vi "pid-auto-tune.vi"() -> ()   [LabVIEW 2019]
uses:
  <vilib>/Rock Robotics/WPI/ThirdParty/JAS_Junk/TrajLib/TypeDef/PID_CONTROLLER.ctl
  <vilib>/Rock Robotics/WPI/ThirdParty/JAS_Junk/TrajLib/LinearFilter_ResetToValue.vi
  <vilib>/Rock Robotics/WPI/ThirdParty/JAS_Junk/TrajLib/LinearFilter_Calculate.vi
  <vilib>/Rock Robotics/WPI/ThirdParty/JAS_Junk/TrajLib/MathUtil_Clamp.vi
  <vilib>/Rock Robotics/WPI/ThirdParty/JAS_Junk/TrajLib/SlewRateLimiter_New.vi
  <vilib>/Rock Robotics/WPI/ThirdParty/JAS_Junk/TrajLib/SlewRateLimiter_Reset.vi
  <vilib>/Rock Robotics/WPI/ThirdParty/JAS_Junk/TrajLib/SlewRateLimiter_Calculate.vi
  <vilib>/Rock Robotics/WPI/ThirdParty/JAS_Junk/TrajLib/SlewRateLimiter_SetRate.vi
  <vilib>/Rock Robotics/WPI/ThirdParty/JAS_Junk/TrajLib/PIDController_AtSetpoint.vi
  <vilib>/Rock Robotics/WPI/ThirdParty/JAS_Junk/TrajLib/PIDController_SetPIDF.vi
  <vilib>/Rock Robotics/WPI/ThirdParty/JAS_Junk/TrajLib/PIDController_SetDerivativeFilter.vi
  <vilib>/Rock Robotics/WPI/ThirdParty/JAS_Junk/TrajLib/PIDController_SetIntegratorRange.vi
  <vilib>/Rock Robotics/WPI/ThirdParty/JAS_Junk/TrajLib/PIDController_SetTolerancePandV.vi
  <vilib>/Rock Robotics/WPI/ThirdParty/JAS_Junk/TrajLib/PIDController_DisableContinousInput.vi
  <vilib>/Rock Robotics/WPI/ThirdParty/JAS_Junk/TrajLib/PIDController_EnableContinousInput.vi
  <vilib>/Rock Robotics/WPI/ThirdParty/JAS_Junk/TrajLib/PIDController_Reset.vi
  <vilib>/Rock Robotics/WPI/ThirdParty/JAS_Junk/TrajLib/PIDController_New.vi
  <vilib>/Rock Robotics/WPI/ThirdParty/JAS_Junk/TrajLib/PIDController_SetOutputLimits.vi
  <vilib>/Rock Robotics/WPI/ThirdParty/JAS_Junk/TrajLib/PIDController_NewPeriod.vi
  <vilib>/Rock Robotics/SystemInterfaces/NetworkCommunication/NetComm_UsageReport_report.vi
  <vilib>/Rock Robotics/WPI/ThirdParty/JAS_Junk/TrajLib/Util_LibraryGlobals.vi
  <vilib>/Rock Robotics/WPI/ThirdParty/JAS_Junk/TrajLib/PIDController_AdvCalculate_FF_Sp_Pv.vi
  <vilib>/addons/control/pid/pid.llb/PID Lead-Lag (DBL).vi
  <vilib>/Rock Robotics/WPI/ThirdParty/JAS_Junk/TrajLib/LinearFilter_MovingAverage.vi
  <vilib>/Rock Robotics/WPI/ThirdParty/JAS_Junk/TrajLib/LinearFilter_LowPassBW1.vi
  <vilib>/Rock Robotics/WPI/ThirdParty/JAS_Junk/TrajLib/LinearFilter_LowPassBW2.vi
  <vilib>/Rock Robotics/WPI/ThirdParty/JAS_Junk/TrajLib/LinearFilter_HighPassBW1.vi
  <vilib>/Rock Robotics/WPI/ThirdParty/JAS_Junk/TrajLib/LinearFilter_HighPassBW2.vi
  <vilib>/addons/control/pid/NI_PID_pid.lvlib
  <vilib>/Rock Robotics/WPI/ThirdParty/JAS_Junk/TrajLib/Trajectory_Library.lvlib
panel:
  out "Plant and Test Data":T1
  out "Tuning Done":bool
  in  "Type of Controller":enum16{"P", "PI", "PID"}(ring)=enum."PI"
  in  "Controller Constant Type":T2(ring)=enum."Ziegler Nicols - Slow"
  in  "Procedure Type":enum16{"Open Loop Step", "Closed Loop Step"}(ring)
  out "New Tuning Parameters":T3
  out "Error Occured":bool
  in  "Tune":bool
  in  "CO Offset":dbl=0.25 format="%#_13g"
  out "Diagnostic Info":T4
  in  "Desired Speed":dbl(slide)=-0.22222222222222499 scale=-10.0..10.0 scale format="%#.1f"
  in  "Tab Control":T5(tab)
  in  "Enable Noise":bool=TRUE
  in  "Auto / Manual":bool=TRUE
  out "Dash Speed Demand":dbl format="%10.2f"
  out "Dash Speed Target":dbl format="%10.2f"
  out "DashLeft Wheel Speed":dbl(knob)=-2.895988890827539e-05 scale=-60.0..60.0
  out "Left Wheel ErrorFilt":dbl format="%11.3f"
  out "DashLeftMotorOutput":dbl format="%11.3f"
  out "Left Wheel Speed Filt":dbl format="%10.2f"
  out "Duration":dbl format="%11.3f"
  out "Late":dbl format="%11.3f"
  out "SP, PV, CO Left":T6(graph)
  in  "SetPoint Change Rate":dbl=80.0 min=1.0 max=9000.0 format="%14.4f"
  in  "Left Adv PID Limits":T7={"MaxInput"=50.0, "MinInput"=-50.0, "Continuous"=FALSE, "MaxOutput"=1.0, "MinOutput"=-1.0}
  in  "Left PID Error Tolerance":T8={"PositionTolerance"=0.001, "VelocityTolerance"=9.9e+30}
  in  "Left Adv PID Tuning":T9={"Kf"=0.02, "Kp"=0.06, "Ki"=0.1, "Kd"=0.004, "MaximumIntegral"=9.9e+30, "MinimumIntegral"=-9.9e+30, "Filter Derivative"=TRUE}
  out "Left PID Data":T10={"Kp"=0.0, "Ki"=0.0, "Kd"=0.0, "Period"=0.0, "Max_Integral"=0.0, "Min_Integral"=0.0, "Max_Input"=0.0, "Min_Input"=0.0, "Continuous"=FALSE, "PositionError"=0.0, "VelocityError"=0.0, "PrevError"=0.0, "TotalError"=0.0, "PositionTolerance"=0.0, "VelocityTolerance"=0.0, "SetPoint"=0.0, "Kf"=0.0, "Prev_Deriv"=0.0, "Prev_Deriv 2"=0.0, "DerivativeFilter"=FALSE, "Min_Output"=-9.99e+35, "Max_Output"=9.9e+35, "Prev_F_P"=0.0, "Prev_F_P_2"=0.0, "AntiWindupActive"=FALSE, "Measurement"=0.0} {"Measurement" format="%16_6e"; "Prev_F_P_2" format="%16_6e"; "Prev_F_P" format="%16_6e"; "Max_Output" format="%16_6e"; "Min_Output" format="%16_6e"; "Prev_Deriv 2" format="%16_6e"; "Prev_Deriv" format="%16_6e"; "Kf" format="%16_6e"; "SetPoint" format="%16_6e"; "VelocityTolerance" format="%16_6e"; "PositionTolerance" format="%16_6e"; "TotalError" format="%16_6e"; "PrevError" format="%16_6e"; "VelocityError" format="%16_6e"; "PositionError" format="%16_6e"; "Min_Input" format="%16_6e"; "Max_Input" format="%16_6e"; "Min_Integral" format="%16_6e"; "Max_Integral" format="%16_6e"; "Period" format="%16_6e"; "Kd" format="%16_6e"; "Ki" format="%16_6e"; "Kp" format="%16_6e"}
  in  "LeftWheelNoise":dbl
  out "LeftWheelSpeed":dbl
  out "LeftMotorOutput":dbl
  out "SpeedSetpoint":dbl
  in  "SpeedTarget":dbl
  in  "SpeedControlEnabled":bool
  out "LibUsage_Kinematics":i32 format="%20.0f"
  out "LibUsage_TrapezoidProfile":i32 format="%20.0f"
  out "LibUsage_LinearFIlter":i32 format="%20.0f"
  out "LibUsage_Odometry":i32 format="%20.0f"
  out "LibUsage_PIDController":i32 format="%20.0f"
  out "LibUsage_ProfiledPID":i32 format="%20.0f"
  # "Enter a desired speed and then press the Set Speed Target \nbutton.  This simulates the joystick input."
  # "FT/SEC"
  # "Example of Closed Loop Motor Speed Control\nUses Advanced PID"
  # "This value shows the current speed of each wheel.  This is measured by an encoder.  The encoder measures\n speed by counting pulses of the wheel turning and dividing by the time interval.  Total distance change\nis also a result.  This value is called the \"Process Variable\"."
  # "FT/SEC"
  # "FT/SEC"
  # "The Speed Target is rate limited so not to make\nto drastic a change in the desired speed.  (This is\nwhat happens mechanically when pushing the gas\npedal of a real car.)"
  # "This error value shows the error between the current speed\nand the speed demand."
  # "FT/SEC"
  # "This example adds a \"Manual\" mode so that the still operates\nif the encoder fails."
  # "FT/SEC"
  # "This value shows the current motor output demand.  This could also be a motor speed demand and \nanother closed loop controller would control the motor speed.  In this simple example this value is \nused to drive the simulated motor directly.  This motor demand is called the \"Control Output\"."
  # "Enables some simulated process noise"
  # "FT/SEC/SEC"
  # "These are the tuning parameters for the PID VI"
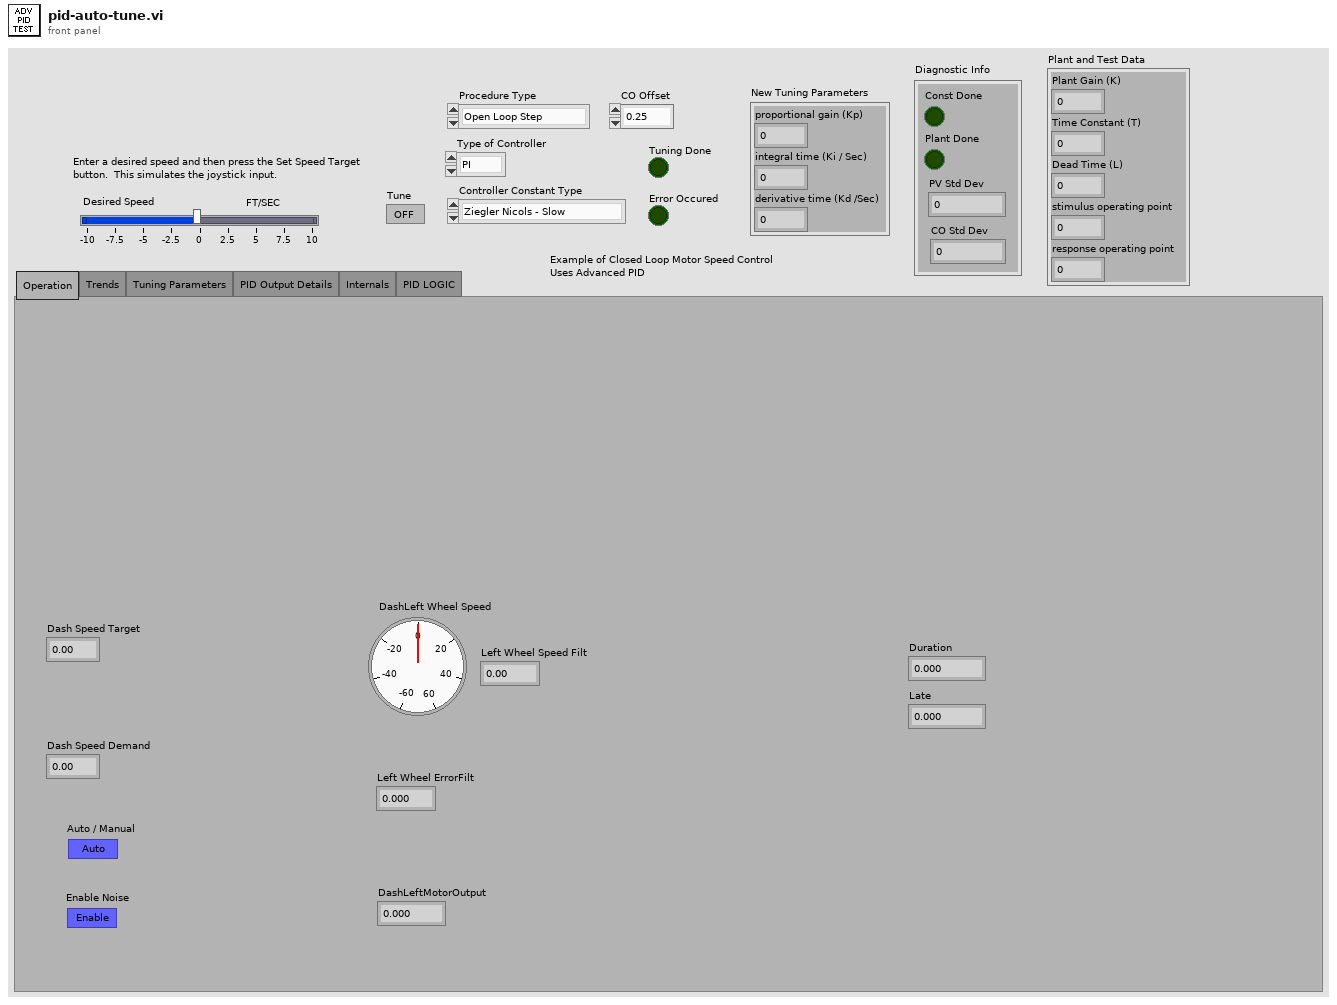
[diagram p1: front panel]
types:
  T1 = cluster{"Plant Gain (K)":dbl, "Time Constant (T)":dbl, "Dead Time (L)":dbl, "stimulus operating point":dbl, "response operating point":dbl}
  T2 = enum16{"Ziegler Nicols - Fast", "Ziegler Nicols - Normal", "Ziegler Nicols - Slow", "CHR regulator - 0% overshoot", "CHR regulator - 20% overshoot", "CHR servo - 0 % overshoot", "CHR servo - 20% overshoot"}
  T3 = cluster{"proportional gain (Kp)":dbl, "integral time (Ki / Sec)":dbl, "derivative time (Kd /Sec)":dbl}
  T4 = cluster{"Const Done":bool, "Plant Done":bool, "PV Std Dev":dbl, "CO Std Dev":dbl}
  T5 = enum32{"Operation", "Trends", "Tuning Parameters", "PID Output Details", "Internals", "PID LOGIC"}
  T6 = cluster{"MotorDemand":dbl, "CurrentSetpoint":dbl, "CurrentPosition":dbl}
  T7 = cluster{"MaxInput":dbl, "MinInput":dbl, "Continuous":bool, "MaxOutput":dbl, "MinOutput":dbl}
  T8 = cluster{"PositionTolerance":dbl, "VelocityTolerance":dbl}
  T9 = cluster{"Kf":dbl, "Kp":dbl, "Ki":dbl, "Kd":dbl, "MaximumIntegral":dbl, "MinimumIntegral":dbl, "Filter Derivative":bool}
  T10 = typedef "Trajectory_Library.lvlib/PID_CONTROLLER.ctl" = cluster{"Kp":dbl, "Ki":dbl, "Kd":dbl, "Period":dbl, "Max_Integral":dbl, "Min_Integral":dbl, "Max_Input":dbl, "Min_Input":dbl, "Continuous":bool, "PositionError":dbl, "VelocityError":dbl, "PrevError":dbl, "TotalError":dbl, "PositionTolerance":dbl, "VelocityTolerance":dbl, "SetPoint":dbl, "Kf":dbl, "Prev_Deriv":dbl, "Prev_Deriv 2":dbl, "DerivativeFilter":bool, "Min_Output":dbl, "Max_Output":dbl, "Prev_F_P":dbl, "Prev_F_P_2":dbl, "AntiWindupActive":bool, "Measurement":dbl}
  T11 = cluster{"gain":dbl, "lag time":dbl, "lead time":dbl}
  T12 = enum16{"Moving Average", "Low Pass 1st Order Butterworth", "Low Pass 2nd Order Butterworth", "High Pass 1st Order Butterworth", "High Pass 2nd Order Butterworth"}
  T13 = cluster{"LeftMotorOutput":dbl, "SpeedSetpoint":dbl, "LeftWheelSpeed":dbl}
  T14 = cluster{"Controller Constant Type":enum16{"Ziegler Nicols - Fast", "Ziegler Nicols - Normal", "Ziegler Nicols - Slow", "CHR regulator - 0% overshoot", "CHR regulator - 20% overshoot", "CHR servo - 0 % overshoot", "CHR servo - 20% overshoot"}, "Type of Controller":enum16{"P", "PI", "PID"}, "CO Offset":dbl, "Kn":dbl, "Tuning Tolerance":dbl, "Plant Tolerance":dbl, "Newest Avg Time ":i32, "Long Ave Time":i32}
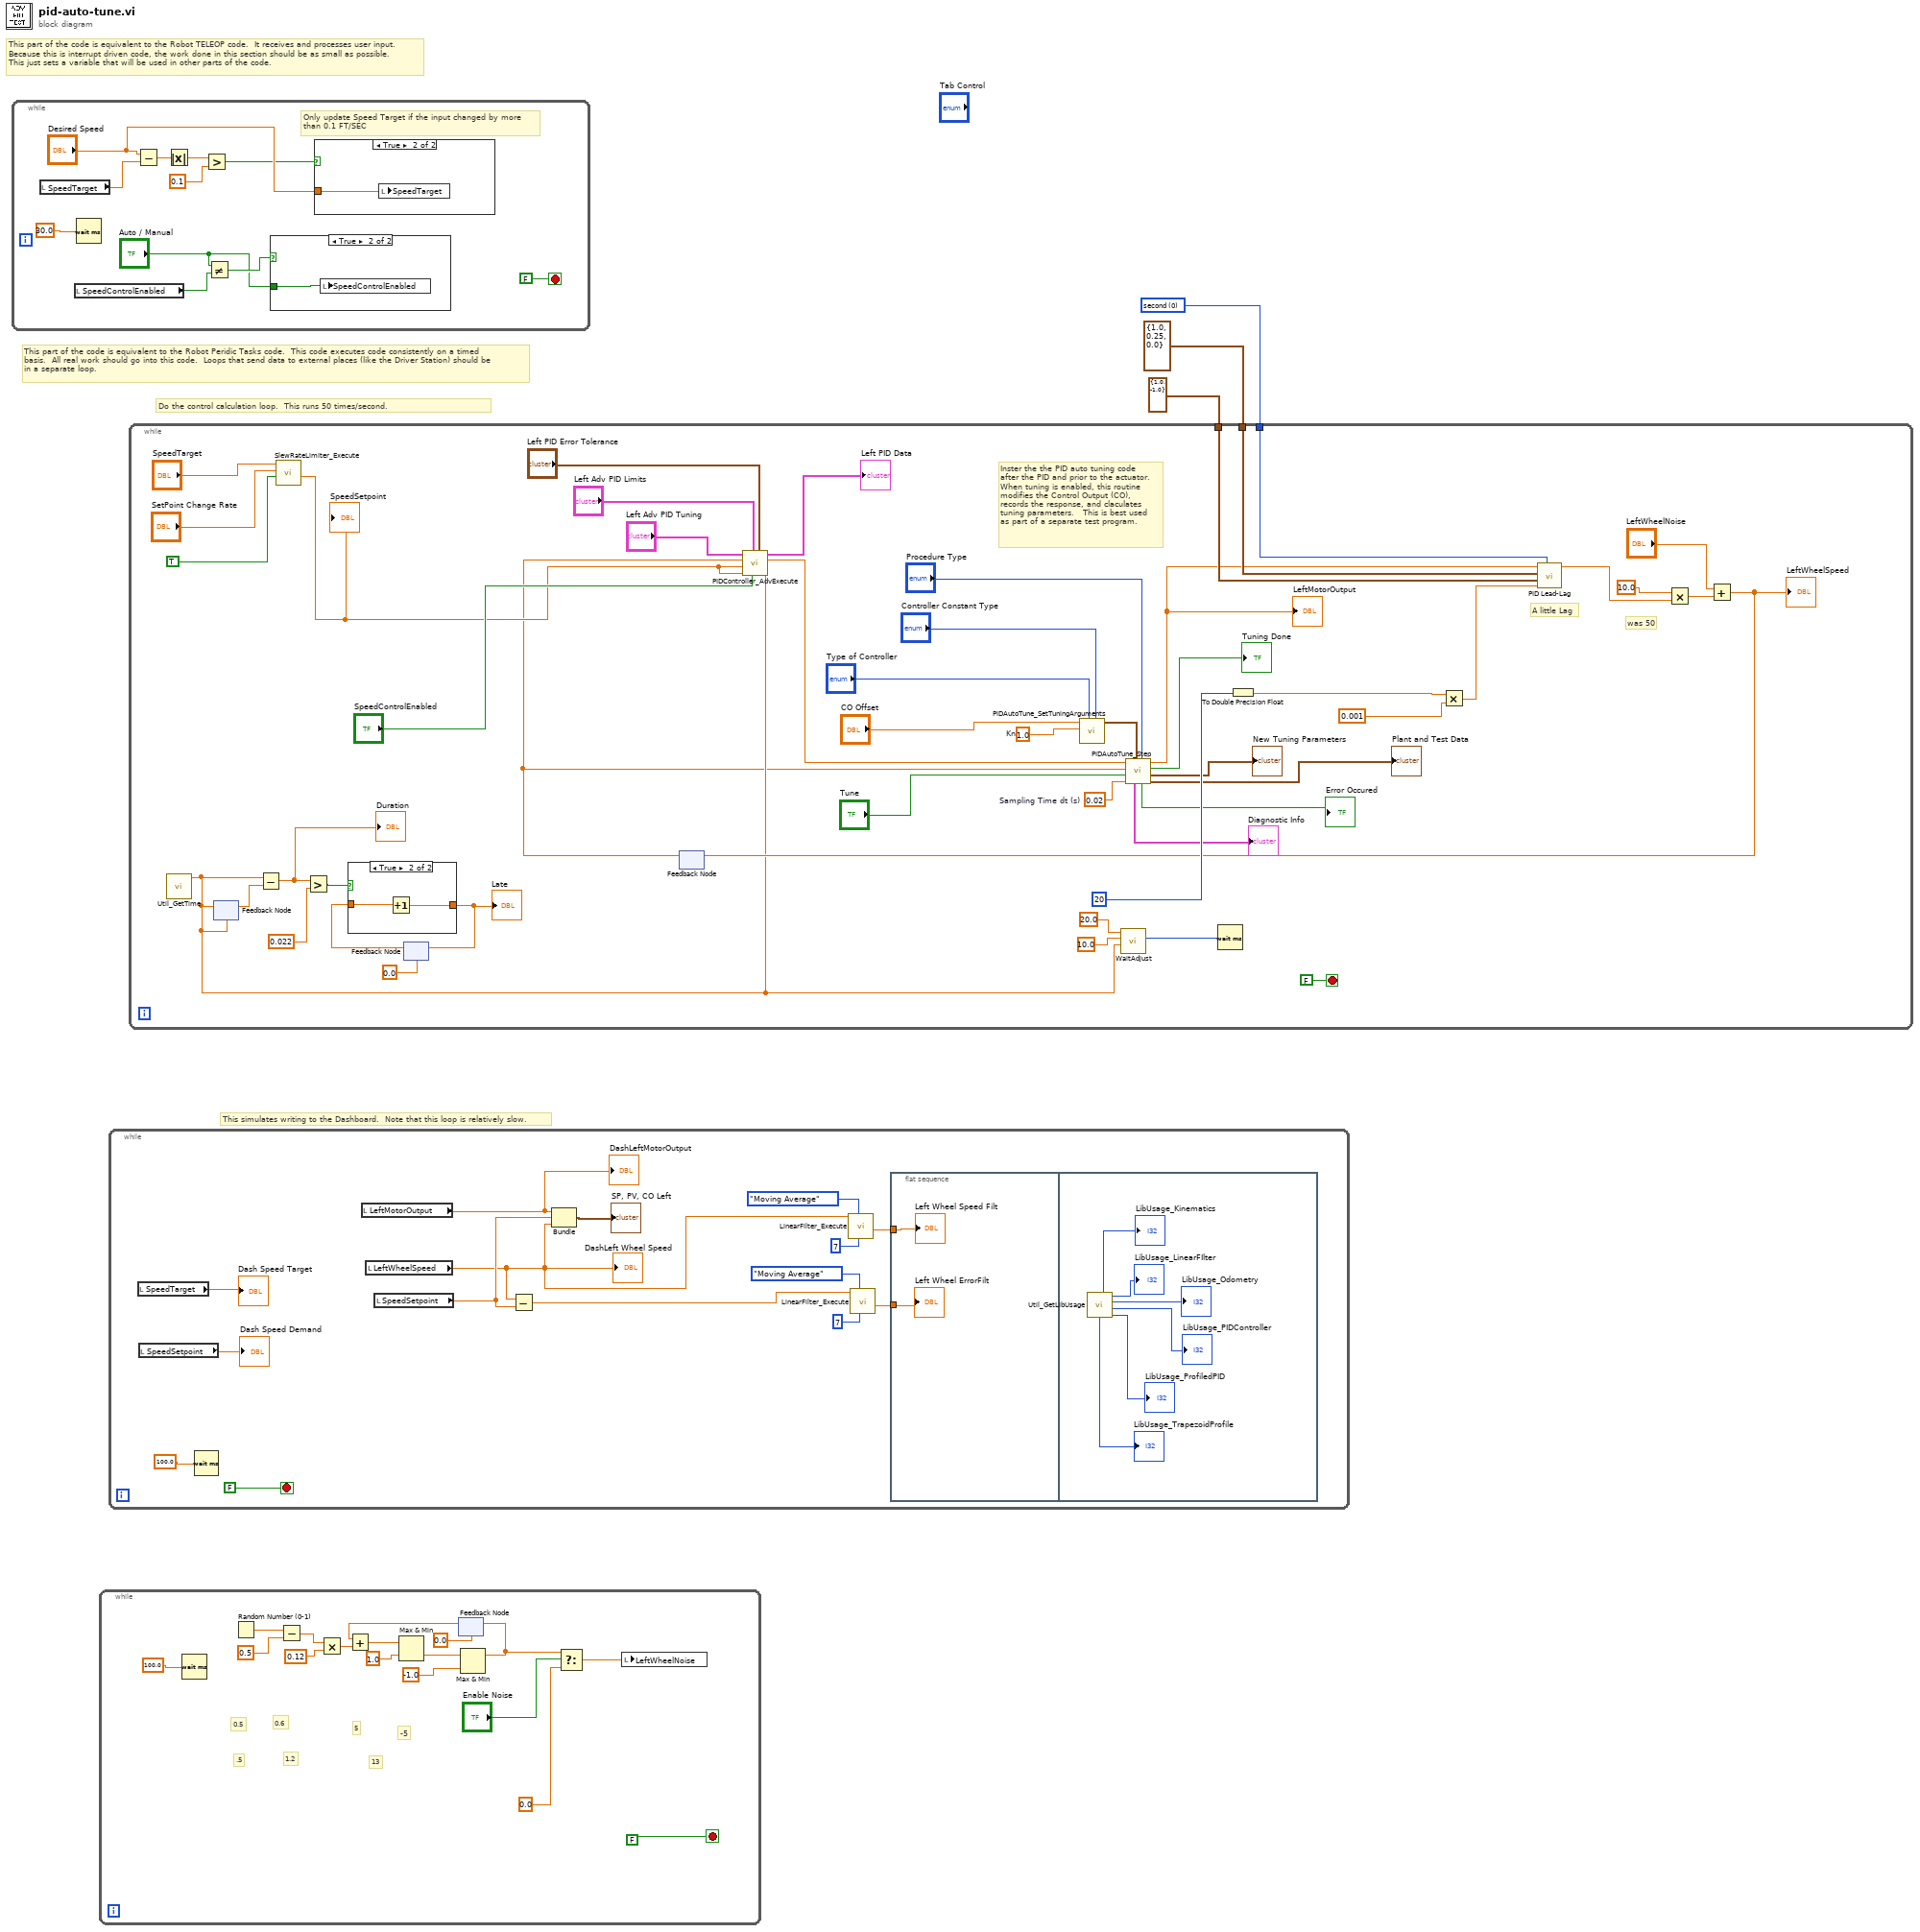
[diagram p0: block diagram]
diagram:
  w3 = u16 0 items=["second", "minute"] ("time unit")
  # "This simulates writing to the Dashboard.  Note that this loop is relatively slow."
  # "Do the control calculation loop.  This runs 50 times/second."
  # "This part of the code is equivalent to the Robot Peridic Tasks code.  This code executes code consistently on a timed\nbasis.  All real work should go into this code.  Loops that send data to external places (like the Driver Station) should be \nin a separate loop."
  # "This part of the code is equivalent to the Robot TELEOP code.  It receives and processes user input.\nBecause this is interrupt driven code, the work done in this section should be as small as possible.\nThis just sets a variable that will be used in other parts of the code."
  n1 = while {
    stop <- FALSE stop-if-true
    # "Only update Speed Target if the input changed by more\nthan 0.1 FT/SEC"
    n2 = local read "SpeedTarget"() -> (w13:dbl)
    n3 = local read "SpeedControlEnabled"() -> (w5:bool)
    n4 = Wait (ms)(milliseconds to wait=30.0) -> ()  [unwired: 1 out]
    n5 = Subtract(x="Desired Speed", y=w13) -> (x-y=w12:dbl)
    n6 = Absolute Value(x=w12) -> (abs(x)=w11:dbl)
    n7 = Greater?(x=w11, y=0.1) -> (0:w8:bool)
    n8 = Not Equal?(x="Auto / Manual", y=w5) -> (x != y?=w6:bool)
    n9 = case shown="True" w6 {
      tunnel: "Auto / Manual" -> [_ w15]
      frame False {
      }
      frame True {
        n10 = local write "SpeedControlEnabled"(w15) -> ()
      }
    }
    n11 = case shown="True" w8 {
      tunnel: "Desired Speed" -> [_ w16]
      frame False {
      }
      frame True {
        n12 = local write "SpeedTarget"(w16) -> ()
      }
    }
  }
  n13 = while {
    stop <- FALSE stop-if-true
    # "-5"
    # "5"
    # "0.6"
    # "0.5"
    # "13"
    # "1.2"
    # ".5"
    n14 = Wait (ms)(milliseconds to wait=100.0) -> ()  [unwired: 1 out]
    n15 = Random Number (0-1)() -> (number: 0 to 1=w17:dbl)
    n16 = Subtract(x=w17, y=0.5) -> (x-y=w24:dbl)
    n17 = Multiply(x=w24, y=0.12) -> (x*y=w23:dbl)
    n18 = feedback #1(0.0) -> (w26:dbl)
    n19 = Add(x=w26, y=w23) -> (x+y=w30:dbl)
    n20 = Max & Min(x=w30, y=1.0) -> (min(x,y)=w29:dbl)  [unwired: 1 out]
    n21 = Max & Min(x=w29, y=-1.0) -> (max(x,y)=w20:dbl)  [unwired: 1 out]
    n22 = feedback-in #1(w20) -> ()
    n23 = Select(t=w20, s="Enable Noise", f=0.0) -> (s? t:f=w21:dbl)
    n24 = local write "LeftWheelNoise"(w21) -> ()
  }
  n25 = while {
    stop <- FALSE stop-if-true
    n26 = local read "SpeedTarget"() -> (→"Dash Speed Target":dbl)
    n27 = local read "SpeedSetpoint"() -> (→"Dash Speed Demand":dbl)
    n28 = Wait (ms)(milliseconds to wait=100.0) -> ()  [unwired: 1 out]
    n29 = local read "LeftMotorOutput"() -> (w43:dbl)
    "DashLeftMotorOutput" <- w43
    n30 = local read "LeftWheelSpeed"() -> (w39:dbl)
    "DashLeft Wheel Speed" <- w39
    n31 = local read "SpeedSetpoint"() -> (w42:dbl)
    n32 = Subtract(x=w39, y=w42) -> (x-y=w35:dbl)
    n33 = Bundle("LeftMotorOutput"=w43, "SpeedSetpoint"=w42, "LeftWheelSpeed"=w39) -> (→"SP, PV, CO Left":T13)  [unwired: 1 in]
    n34 = call <vilib>:"LinearFilter_Execute.vi"("Samples"=7, "Filter Type"=T12."Moving Average", "Input"=w39) -> ("Output"=w38:dbl)  [unwired: 7 in, 1 out]
    n35 = call <vilib>:"LinearFilter_Execute.vi"("Samples"=7, "Filter Type"=T12."Moving Average", "Input"=w35) -> ("Output"=w34:dbl)  [unwired: 7 in, 1 out]
    n36 = flat-sequence {
      tunnel: w38 -> [w50]
      tunnel: w34 -> [w49]
      frame #0 {
        "Left Wheel ErrorFilt" <- w49
        "Left Wheel Speed Filt" <- w50
      }
      frame #1 {
        n37 = call <vilib>:"Util_GetLibUsage.vi"() -> ("LibUsage_ProfiledPID"=→"LibUsage_ProfiledPID":i32, "LibUsage_PIDController"=→"LibUsage_PIDController":i32, "LibUsage_Odometry"=→"LibUsage_Odometry":i32, "LibUsage_LinearFIlter"=→"LibUsage_LinearFIlter":i32, "LibUsage_TrapezoidProfile"=→"LibUsage_TrapezoidProfile":i32, "LibUsage_Kinematics"=→"LibUsage_Kinematics":i32)  [unwired: 6 in]
      }
    }
  }
  n38 = while {
    tunnel: w3 -> [w87]
    tunnel: T11 {"gain"=1.0, "lag time"=0.25, "lead time"=0.0} ("tuning parameters") -> [w86]
    tunnel: cluster{"output high":dbl, "output low":dbl} {"output high"=1.0, "output low"=-1.0} ("output range") -> [w85]
    stop <- FALSE stop-if-true
    w73 = 0.02  # Sampling Time dt (s)
    w72 = 1.0  # Kn
    # "was 50"
    # "Inster the the PID auto tuning code\nafter the PID and prior to the actuator.\nWhen tuning is enabled, this routine\nmodifies the Control Output (CO), \nrecords the response, and claculates\ntuning parameters.   This is best used\nas part of a separate test program."
    # "A little Lag"
    n39 = call <vilib>:"Util_GetTime.vi"() -> ("FPGA_Time_Seconds"=w74:dbl)  [unwired: 10 in, 1 out]
    n40 = feedback #2(w74) -> (w99:dbl)
    n41 = feedback-in #2(w74) -> ()
    n42 = Subtract(x=w74, y=w99) -> (x-y=w97:dbl)
    "Duration" <- w97
    n43 = call <vilib>:"SlewRateLimiter_Execute.vi"("Enable"=TRUE, "Rate"="SetPoint Change Rate", "Input"="SpeedTarget") -> ("Output"=w80:dbl)  [unwired: 7 in, 1 out]
    "SpeedSetpoint" <- w80
    n44 = Greater?(x=w97, y=0.022) -> (0:w98:bool)
    n45 = feedback #3(0.0) -> (w100:dbl)
    n46 = case shown="True" w98 {
      tunnel: [w106 w108] -> w101
      tunnel: w100 -> [w106 w107]
      frame False {
      }
      frame True {
        n47 = Increment(x=w107) -> (x+1=w108:dbl)
      }
    }
    "Late" <- w101
    n48 = feedback-in #3(w101) -> ()
    n49 = feedback #4() -> (w64:dbl)  [unwired: 1 in]
    n50 = call <vilib>:"PIDController_AdvExecute.vi"("Time"=w74, "PID Error Tolerance"="Left PID Error Tolerance", "Auto"="SpeedControlEnabled", "Adv PID Limits"="Left Adv PID Limits", "FF-FeedForward"=w80, "SP-SetPoint"=w80, "PV-Measurement"=w64, "Adv PID Tuning"="Left Adv PID Tuning") -> ("CO-ControlOutput"=w65:dbl, "out PID_CONTROLLER"=→"Left PID Data":T10)  [unwired: 1 in, 1 out]
    n51 = call <vilib>:"PIDAutoTune_SetTuningArguments.vi"("Controller Constant Type"="Controller Constant Type", "Type of Controller"="Type of Controller", "Kn"=w72, "CO Offset"="CO Offset") -> ("Configuration Parameters"=w67:T14)  [unwired: 7 in]
    n52 = call <vilib>:"WaitAdjust.vi"("Time_SEC"=w74, "MaxDeviation_MS"=10.0, "DesiredLoopTime_MS"=20.0) -> ("AdjustedWaitTime_MS"=w75:u32)  [unwired: 7 in, 1 out]
    n53 = call <vilib>:"PIDAutoTune_Step.vi"("Procedure Type"="Procedure Type", "Configuration Parameters"=w67, "Sampling Time dt (s)"=w73, "Tune"="Tune", "Measurement  (PV)"=w64, "Control Output (Co)"=w65) -> ("Plant and Test Data"=→"Plant and Test Data":T1, "New Tuning Parameters"=→"New Tuning Parameters":T3, "Tuning Done"=→"Tuning Done":bool, "Adj CO"=w66:dbl, "Error Occured"=→"Error Occured":bool, "Diagnostic Info"=→"Diagnostic Info":T4)
    "LeftMotorOutput" <- w66
    n54 = Wait (ms)(milliseconds to wait=w75) -> ()  [unwired: 1 out]
    n55 = To Double Precision Float(number=u32 20 ("milliseconds to wait")) -> (double precision float=w83:dbl)
    n56 = Multiply(x=w83, y=0.001) -> (x*y=w92:dbl)
    n57 = call-poly <vilib>:"PID Lead-Lag.vi"("time unit"=w87, "dt (s)"=w92, "output range"=w85, "tuning parameters"=w86, "input"=w66) -> ("output"=w93:dbl)  [unwired: 3 in, 1 out]
    n58 = Multiply(x=10.0, y=w93) -> (x*y=w90:dbl)
    n59 = Add(x="LeftWheelNoise", y=w90) -> (x+y=w82:dbl)
    "LeftWheelSpeed" <- w82
    n60 = feedback-in #4(w82) -> ()
  }
